vi "ShowData.vi"(11 "messengerMbase in":refnum<class "MessengerMBase.lvclass">) -> (0 "abort":bool, 1 "acks":u32[](array[numeric]), 2 "subchannels":T2(array[cluster]), 3 "messengerMbase out":refnum<class "MessengerMBase.lvclass">, 4 "lastID":u32)   [LabVIEW 2019, in "MessengerM.lvlib" / "MessengerMBase.lvclass"]
uses:
  MessengerMBase.lvclass
  Element.ctl
  MessengerM.lvlib
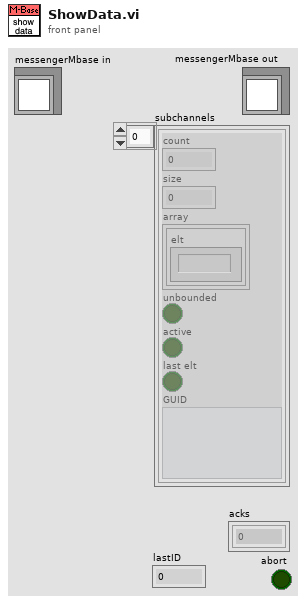
[diagram p1: front panel]
types:
  T1 = typedef "MessengerM.lvlib/Element.ctl" = string
  T2 = cluster{"count":i32, "size":i32, "array":cluster{"elt":T1}[], "unbounded":bool, "active":bool, "last elt":bool, "GUID":string}[]
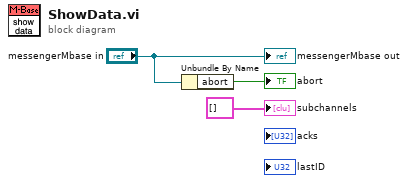
[diagram p0: block diagram]
diagram:
  n1 = Unbundle By Name("messengerMbase in") -> ("abort"=→"abort":bool)
  "messengerMbase out" <- "messengerMbase in"
  "subchannels" <- T2 [] ("subchannels")
